vi "getTravelRange.vi"(11 "EEPROM_string":string) -> (0 "error out":errorcluster, 3 "travelRange":cluster{"X":dbl, "Y":dbl, "Z":dbl})   [LabVIEW 2015]
uses:
  flipYZdbl.vi
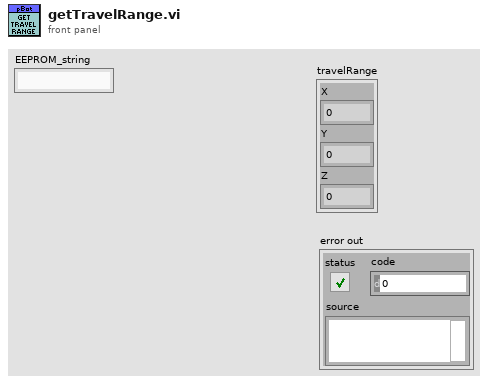
[diagram p1: front panel]
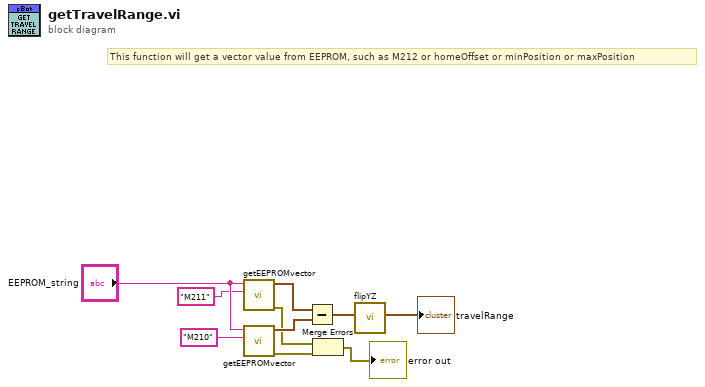
[diagram p0: block diagram]
diagram:
  # "This function will get a vector value from EEPROM, such as M212 or homeOffset or minPosition or maxPosition"
  n1 = call "getEEPROMvector.vi"("vectorName"="M211", "EEPROM_Settings"="EEPROM_string") -> ("error out"=w5:errorcluster, "vectorOut"=w7:cluster{dbl, dbl, dbl})  [unwired: 8 in]
  n2 = call "getEEPROMvector.vi"("vectorName"="M210", "EEPROM_Settings"="EEPROM_string") -> ("error out"=w4:errorcluster, "vectorOut"=w6:cluster{dbl, dbl, dbl})  [unwired: 8 in]
  n3 = Subtract(x=w7, y=w6) -> (x-y=w2:cluster{dbl, dbl, dbl})
  n4 = Merge Errors(w5, w4) -> (→"error out":errorcluster)
  n5 = call-poly "flipYZ.vi"("pointIn"=w2) -> ("pointOut"=→"travelRange":cluster{"X":dbl, "Y":dbl, "Z":dbl})  [unwired: 10 in]
